vi "get extern command 3.vi"() -> (1 "aux (U24)":u32, 2 "extern command":T1, 3 "valid command?":bool)   [LabVIEW 2019]
uses:
  extern commands 3.ctl
  <vilib>/rvi/interface/RandomDataEmulation/niFpgaRandomDataHandleErrors.vi
  <vilib>/rvi/DataTransferAndStorage/Container/XNode/niFpgaContainer.xnode
  <vilib>/rvi/interface/RandomDataEmulation/nirviRandomDataFpgaReadWriteTemplate.vi
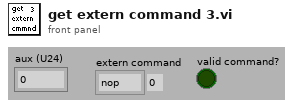
[diagram p1: front panel]
types:
  T1 = typedef "extern commands 3.ctl" = enum8{"nop", "dly", "wfm", "prog", "stop", "wait"}
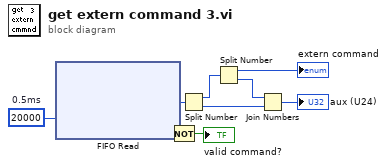
[diagram p0: block diagram]
diagram:
  w4 = 20000  # 0.5ms
  n1 = xnode ("FIFO Read")("Timeout"=w4) -> ("Element"=w3:u32, "Timed Out?"=w2:bool)  [unwired: 1 in, 1 out]
  n2 = Not(x=w2) -> (.not. x?=→"valid command?":bool)
  n3 = Split Number(x=w3) -> (hi(x)=w6:u16, lo(x)=w8:u16)
  n4 = Split Number(x=w6) -> (hi(x)=→"extern command":u8, lo(x)=w7:u8)
  n5 = Join Numbers(hi=w7, lo=w8) -> ((hi.lo)=→"aux (U24)":u32)
